vi "FastMap - Update View.vi"(8 "Column":i32, 9 "Row":i32, 10 "View":i32[](array[numeric]) caption="View (-1 team, 0 empty, 1 enemy)", 11 "fast map in":refnum<data-value>) -> (3 "fast map out":refnum<data-value>)   [LabVIEW 2015, in "DS Square.lvlib"]
uses:
  DS Square.lvlib
  Common/Common.lvlib
  Common/Position.ctl
  Square/Square.lvclass
  Square State Fast.ctl
  Fast Map.ctl
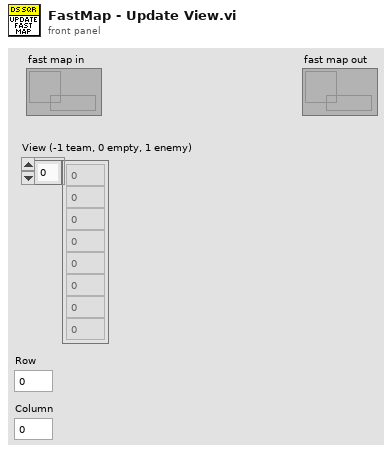
[diagram p1: front panel]
types:
  T1 = typedef "Common.lvlib/Position.ctl" = cluster{"Column":i32, "Row":i32}
  T2 = typedef "DS Square.lvlib/Square State Fast.ctl" = enum8{"Unknown", "Empty", "Occupied - Active", "Occupied - Cool Down", "Attacked", "Enemy", "Enemy Wall"}
  T3 = typedef "DS Square.lvlib/Fast Map.ctl" = cluster{"state":T2[][], "updated":i32[][]}
  T4 = typedef "SB Type Defs.lvlib/Direction Enum.ctl" = enum16{"NW", "N", "NE", "E", "SE", "S", "SW", "W"}
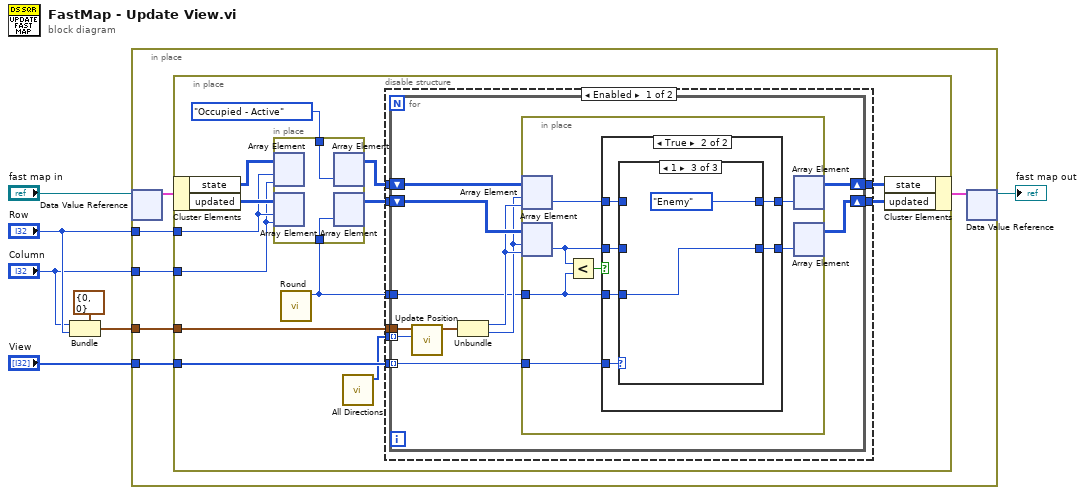
[diagram p0: block diagram]
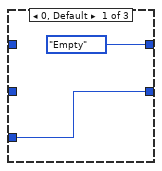
[diagram p3: hidden frame]
diagram:
  n1 = Bundle(cluster=T1 {"Column"=0, "Row"=0} ("Position in"), "Column"="Column", "Row"="Row") -> (w1:T1)
  n2 = in-place {
    in-place-border: "View" -> [w11]
    in-place-border: w1 -> [w12]
    in-place-border: "Row" -> [w9]
    in-place-border: "Column" -> [w8]
    n3 = in-place-dvr #1("fast map in") -> (w13:T3)  [unwired: 1 out]
    n4 = in-place {
      in-place-border: w12 -> [w24]
      in-place-border: w11 -> [w23]
      in-place-border: w9 -> [w18]
      in-place-border: w8 -> [w17]
      n5 = in-place-cluster #2(w13) -> ("state"=w21:T2[][], "updated"=w22:i32[][])
      n6 = call "Round.vi"() -> ("Round"=w16:i32)  [unwired: 11 in]
      n7 = in-place {
        in-place-border: w16 -> [w70]
        in-place-border: Square_State_Fast."Occupied - Active" ("element") -> [w69]
        n8 = in-place-array #3(w21, w18, w17) -> ()  [unwired: 1 out]
        n9 = in-place-array #4(w22, w18, w17) -> ()  [unwired: 1 out]
        n10 = in-place-array #3(w69) -> (w19:T2[][])  [unwired: 2 out]
        n11 = in-place-array #4(w70) -> (w20:i32[][])  [unwired: 2 out]
      }
      n12 = call "All Directions.vi"() -> ("All directions"=w14:T4[])  [unwired: 11 in]
      n13 = disable-structure shown="Enabled" {
        disable-tunnel: [w34 w68] -> w26
        disable-tunnel: [w33 w67] -> w25
        disable-tunnel: w24 -> [w32 _]
        disable-tunnel: w23 -> [w31 _]
        disable-tunnel: w20 -> [w30 w67]
        disable-tunnel: w19 -> [w29 w68]
        disable-tunnel: w16 -> [w28 _]
        disable-tunnel: w14 -> [w27 _]
        frame Enabled {
          n14 = for {
            tunnel: w31 -> [w44] mode=indexing
            shift-right: [w43] -> w34
            shift-left: w29 -> [w45]
            tunnel: w32 -> [w37]
            shift-right: [w39] -> w33
            shift-left: w30 -> [w42]
            tunnel: w28 -> [w38]
            tunnel: w27 -> [w35] mode=indexing
            n15 = call "Update Position.vi"("Direction"=w35, "Position in"=w37) -> ("Position out"=w36:T1)  [unwired: 9 in]
            n16 = Unbundle(w36) -> ("Column"=w41:i32, "Row"=w40:i32)
            n17 = in-place {
              in-place-border: w44 -> [w52]
              in-place-border: w38 -> [w46]
              n18 = in-place-array #5(w45, w40, w41) -> (w51:T2)
              n19 = in-place-array #6(w42, w40, w41) -> (w48:i32)
              n20 = Less?(x=w48, y=w46) -> (x < y?=w50:bool)
              n21 = case shown="True" w50 {
                tunnel: w52 -> [_ w60]
                tunnel: w51 -> [w54 w59]
                tunnel: [w54 w58] -> w49
                tunnel: w48 -> [w53 w57]
                tunnel: w46 -> [_ w56]
                tunnel: [w53 w55] -> w47
                frame False {
                  # "already updated this round"
                }
                frame True {
                  n22 = case shown="1" w60 {
                    tunnel: w59 -> [_ w64 _]
                    tunnel: [Square_State_Fast."Empty" ("element") w64 Square_State_Fast."Enemy" ("element")] -> w58
                    tunnel: w57 -> [_ w63 _]
                    tunnel: w56 -> [w61 _ w65]
                    tunnel: [w61 w63 w65] -> w55
                    frame 0, Default {
                    }
                    frame -1 {
                      # "don't update this...\nlast update indicates\nhow much longer cool\ndown will last"
                    }
                    frame 1 {
                    }
                  }
                }
              }
              n23 = in-place-array #5(w49) -> (w43:T2[][])  [unwired: 2 out]
              n24 = in-place-array #6(w47) -> (w39:i32[][])  [unwired: 2 out]
            }
          }
        }
        frame Disabled {
        }
      }
      n25 = in-place-cluster #2("state"=w26, "updated"=w25) -> (w10:T3)
    }
    n26 = in-place-dvr #1(w10) -> (→"fast map out":refnum<data-value>)  [unwired: 1 out]
  }
